vi "Disable Enable Controls.vi"(10 "Disable or Enable":T1(ring), 11 "Cluster":T2) -> (0 "error out":errorcluster)   [LabVIEW 2025]
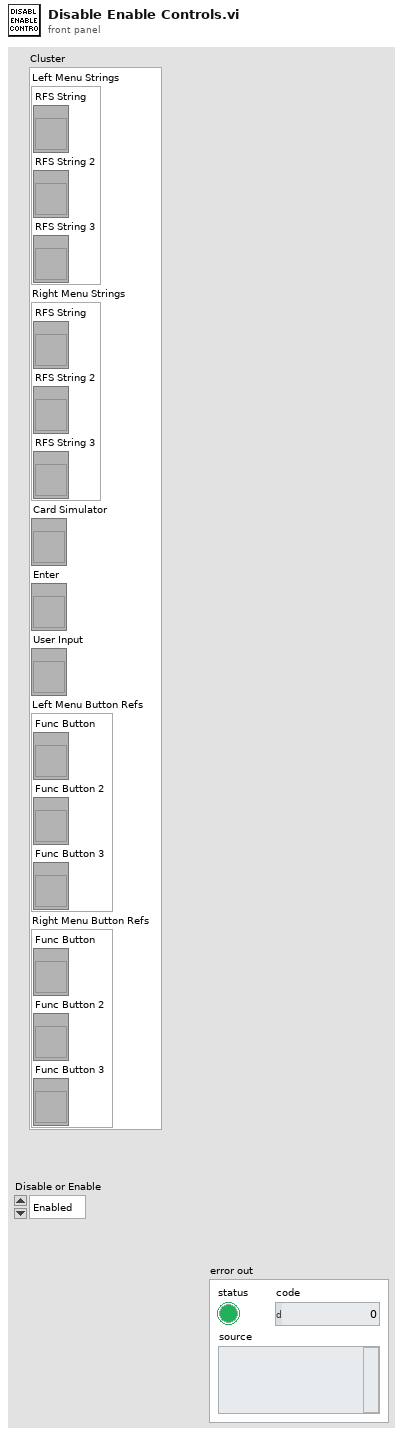
[diagram p1: front panel]
types:
  T1 = enum8{"Enabled", "Disabled", "Disabled and Grayed Out"}
  T2 = cluster{"Left Menu Strings":cluster{"RFS String":refnum<vi>, "RFS String 2":refnum<vi>, "RFS String 3":refnum<vi>}, "Right Menu Strings":cluster{"RFS String":refnum<vi>, "RFS String 2":refnum<vi>, "RFS String 3":refnum<vi>}, "Card Simulator":refnum<vi>, "Enter":refnum<vi>, "User Input":refnum<vi>, "Left Menu Button Refs":cluster{"Func Button":refnum<vi>, "Func Button 2":refnum<vi>, "Func Button 3":refnum<vi>}, "Right Menu Button Refs":cluster{"Func Button":refnum<vi>, "Func Button 2":refnum<vi>, "Func Button 3":refnum<vi>}}
  T3 = cluster{"Func Button":refnum<vi>, "Func Button 2":refnum<vi>, "Func Button 3":refnum<vi>}
  T4 = cluster{"RFS String":refnum<vi>, "RFS String 2":refnum<vi>, "RFS String 3":refnum<vi>}
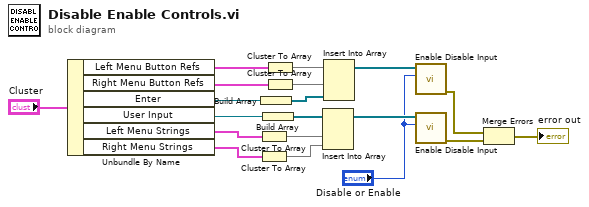
[diagram p0: block diagram]
diagram:
  n1 = Unbundle By Name("Cluster") -> ("Left Menu Button Refs"=w4:T3, "Right Menu Button Refs"=w5:T3, "Enter"=w10:refnum<vi>, "User Input"=w12:refnum<vi>, "Left Menu Strings"=w13:T4, "Right Menu Strings"=w16:T4)
  n2 = Cluster To Array(cluster=w13) -> (array=w15:refnum<vi>[])
  n3 = Cluster To Array(cluster=w16) -> (array=w17:refnum<vi>[])
  n4 = Build Array(w10) -> (w9:refnum<vi>[])
  n5 = Build Array(w12) -> (w14:refnum<vi>[])
  n6 = Cluster To Array(cluster=w4) -> (array=w7:refnum<vi>[])
  n7 = Cluster To Array(cluster=w5) -> (array=w8:refnum<vi>[])
  n8 = Insert Into Array(array=w14, new element #1=w15, new element #2=w17) -> (w18:refnum<vi>[])  [unwired: 1 in]
  n9 = Insert Into Array(array=w7, new element #1=w8, new element #2=w9) -> (w6:refnum<vi>[])  [unwired: 1 in]
  n10 = call "Enable Disable Input.vi"("Disabled"="Disable or Enable", "Input Refs"=w6) -> ("error out"=w3:errorcluster)  [unwired: 9 in]
  n11 = call "Enable Disable Input.vi"("Disabled"="Disable or Enable", "Input Refs"=w18) -> ("error out"=w2:errorcluster)  [unwired: 9 in]
  n12 = Merge Errors(w3, w2) -> (→"error out":errorcluster)
